vi "dfd_TF to ZPK.vi"(10 "denominator":dbl[](array[numeric]), 11 "numerator":dbl[](array[numeric])) -> (1 "gain":dbl, 2 "poles":cdb[](array[numeric]), 3 "zeros":cdb[](array[numeric]))   [LabVIEW 2017, in "NI_DigFilterLicensed.lvlib"]
uses:
  <vilib>/addons/Digital Filter Design/NI_DigFilterLicensed.lvlib
  <vilib>/Analysis/polynomials.llb/Polynomial Roots (DBL).vi
  <vilib>/Analysis/NI_AALPro.lvlib
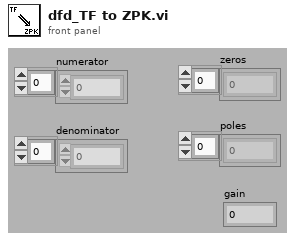
[diagram p1: front panel]
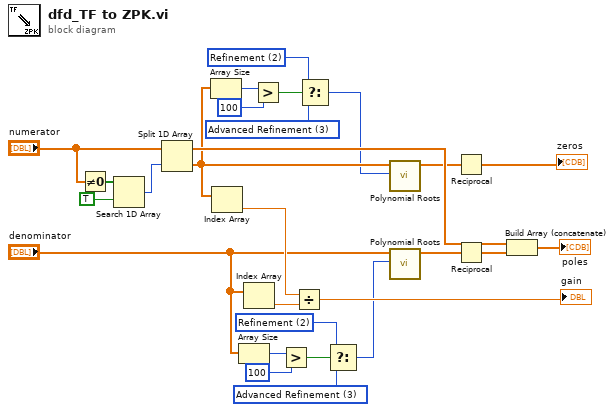
[diagram p0: block diagram]
diagram:
  w7 = u16 3 items=["General", "Simple Classification", "Refinement", "Advanced Refinement"] ("option")
  w2 = u16 2 items=["General", "Simple Classification", "Refinement", "Advanced Refinement"] ("option")
  w9 = u16 3 items=["General", "Simple Classification", "Refinement", "Advanced Refinement"] ("option")
  w10 = u16 2 items=["General", "Simple Classification", "Refinement", "Advanced Refinement"] ("option")
  n1 = Not Equal To 0?(x="numerator") -> (x != 0?=w21:bool[])
  n2 = Search 1D Array(1D array=w21, element=TRUE) -> (index of element=w19:i32)  [unwired: 1 out]
  n3 = Split 1D Array(array="numerator", index=w19) -> (first subarray=w16:dbl[], second subarray=w14:dbl[])
  n4 = Array Size(array=w14) -> (size(s)=w13:i32)
  n5 = Index Array(array=w14) -> (element=w25:dbl)  [unwired: 1 in]
  n6 = Array Size(array="denominator") -> (size(s)=w4:i32)
  n7 = Index Array(array="denominator") -> (element=w26:dbl)  [unwired: 1 in]
  n8 = Greater?(x=w13, y=100) -> (0:w11:bool)
  n9 = Greater?(x=w4, y=100) -> (0:w6:bool)
  n10 = Divide(x=w25, y=w26) -> (x/y=→"gain":dbl)
  n11 = Select(t=w10, s=w11, f=w9) -> (s? t:f=w8:u16)
  n12 = Select(t=w2, s=w6, f=w7) -> (s? t:f=w1:u16)
  n13 = call-poly <vilib>:"Polynomial Roots.vi"("option"=w8, "P(x)"=w14) -> ("Roots"=w15:cdb[])  [unwired: 1 in, 8 out]
  n14 = call-poly <vilib>:"Polynomial Roots.vi"("option"=w1, "P(x)"="denominator") -> ("Roots"=w18:cdb[])  [unwired: 1 in, 8 out]
  n15 = Reciprocal(x=w15) -> (1/x=→"zeros":cdb[])
  n16 = Reciprocal(x=w18) -> (1/x=w23:cdb[])
  n17 = Build Array (concatenate)(w16, w23) -> (→"poles":cdb[])
